vi "Callback - Get Data by Name.vi"(5 "Newest Time to Plot (unix,ns)":u64, 7 "Oldest Time to Plot (unix,ns)":u64, 8 "error in (no error)":errorcluster, 10 "Name":string, 11 "StokePlotHandle in":refnum<class "BjusticePlotHandle.lvclass">) -> (0 "error out":errorcluster, 2 "data history":T1, 3 "StokePlotHandle out":refnum<class "BjusticePlotHandle.lvclass">)   [LabVIEW 2021, in "BjusticePlotHandle.lvclass"]
uses:
  BjusticePlotHandle.lvclass
  TypeDefs/plot datapoint.ctl
  BjusticePlotHandle.lvclass/BjusticePlotHandle.ctl
  e8c38722-4420-420d-a7ba-0e160a98b42c.vi
  e8c38722-4420-420d-a7ba-0e160a98b42c.vi/17d75e1a-130a-47e0-8f2c-6c7d90b8ca77.vi
  <userlib>/bjustice/Ring Buffer for Time Series Data/API Poly.vi
  <userlib>/bjustice/Ring Buffer for Time Series Data/API/Read Full Rotated Buffer.vi
  <userlib>/bjustice/Ring Buffer for Time Series Data Strict Accessor/SubVIs/Search for time to keep.vi
  <userlib>/bjustice/Ring Buffer for Time Series Data Strict Accessor/SubVIs/Index ByteArray.vi
  e8c38722-4420-420d-a7ba-0e160a98b42c.vi/19bdd28a-0674-4be3-87bb-ec701e431d75.vi
  <userlib>/bjustice/Ring Buffer for Time Series Data Strict Accessor/SubVIs/error if empty buffer.vi
  e8c38722-4420-420d-a7ba-0e160a98b42c.vi/17d75e1a-130a-47e0-8f2c-6c7d90b8ca77.vi/bbb64351-fa28-4ac1-b583-44e271193ecd.vi
  <userlib>/bjustice/Ring Buffer for Time Series Data/SubVIs/Rotate Buffer.vi
  <userlib>/bjustice/Ring Buffer for Time Series Data Strict Accessor/SubVIs/Search for oldest time to keep.vi
  <userlib>/bjustice/Ring Buffer for Time Series Data Strict Accessor/SubVIs/Search for newest time to keep.vi
  <userlib>/bjustice/Ring Buffer for Time Series Data Strict Accessor/SubVIs/datatype byte size.vi
  <userlib>/bjustice/Ring Buffer for Time Series Data Strict Accessor/SubVIs/array sizes to number of points.vi
  e8c38722-4420-420d-a7ba-0e160a98b42c.vi/19bdd28a-0674-4be3-87bb-ec701e431d75.vi/81c66277-30bd-484c-9c7c-9646f36721bb.vi
  e8c38722-4420-420d-a7ba-0e160a98b42c.vi/19bdd28a-0674-4be3-87bb-ec701e431d75.vi/7ca10173-70f1-4bfb-9c4b-948090662032.vi
  e8c38722-4420-420d-a7ba-0e160a98b42c.vi/19bdd28a-0674-4be3-87bb-ec701e431d75.vi/ea4aced9-3494-4b3f-b998-02af6afbdac4.vi
  e8c38722-4420-420d-a7ba-0e160a98b42c.vi/19bdd28a-0674-4be3-87bb-ec701e431d75.vi/022c581c-5349-49df-98f9-5a038829ee63.vi
  e8c38722-4420-420d-a7ba-0e160a98b42c.vi/19bdd28a-0674-4be3-87bb-ec701e431d75.vi/ed40bcc8-bbaa-4b61-9e1a-b4b75cf21b06.vi
  e8c38722-4420-420d-a7ba-0e160a98b42c.vi/19bdd28a-0674-4be3-87bb-ec701e431d75.vi/f4b703c2-aaab-40a0-b3da-b0c22dc82d50.vi
  e8c38722-4420-420d-a7ba-0e160a98b42c.vi/19bdd28a-0674-4be3-87bb-ec701e431d75.vi/1efa054f-b143-4d96-9f7e-584a7c6fa7fd.vi
  e8c38722-4420-420d-a7ba-0e160a98b42c.vi/19bdd28a-0674-4be3-87bb-ec701e431d75.vi/b7c29f3f-256a-4401-af9d-aa15374df391.vi
  e8c38722-4420-420d-a7ba-0e160a98b42c.vi/19bdd28a-0674-4be3-87bb-ec701e431d75.vi/2fb7b479-974d-4a18-8674-c4c8d9dc9a89.vi
  e8c38722-4420-420d-a7ba-0e160a98b42c.vi/19bdd28a-0674-4be3-87bb-ec701e431d75.vi/faac7175-5814-4bb6-a961-a8db1f460653.vi
  e8c38722-4420-420d-a7ba-0e160a98b42c.vi/19bdd28a-0674-4be3-87bb-ec701e431d75.vi/b6af2a6f-71a4-4cfe-837f-b196861458b0.vi
  <userlib>/bjustice/Ring Buffer for Time Series Data/SubVIs/Split Values Array.vi
  <userlib>/bjustice/Ring Buffer for Time Series Data/SubVIs/Enforce array size multiple timestamps.vi
  <vilib>/Utility/error.llb/Trim Whitespace.vi
  <vilib>/Utility/error.llb/Error Cluster From Error Code.vi
  RocketPlot.lvlib
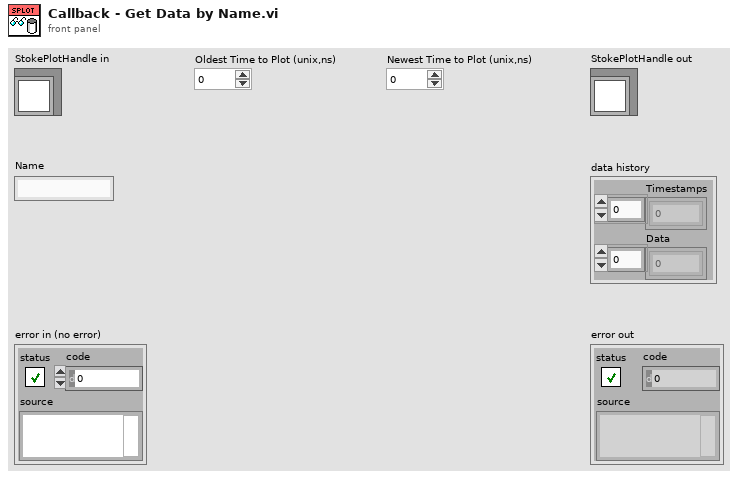
[diagram p1: front panel]
types:
  T1 = typedef "RocketPlot.lvlib/plot datapoint.ctl" = cluster{"Timestamps":u64[], "Data":dbl[]}
  T2 = typedef "Ring Buffer Strict Accessor.lvlib/RingBufferHandle.ctl" = cluster{"Ring buffer DVR":refnum<data-value>, "Data Type":T3, "Size(s)":i32[], "Endianess":T4, "Buffer Size (#timestamps) [init]":i32}
  T3 = typedef "Ring Buffer Strict Accessor.lvlib/DataType.ctl" = enum16{"uint8", "uint16", "uint32", "uint64", "int8", "int16", "int32", "int64", "float", "double", "extended"}
  T4 = typedef "Ring Buffer Strict Accessor.lvlib/Endianess.ctl" = enum16{"big-endian", "little-endian"}
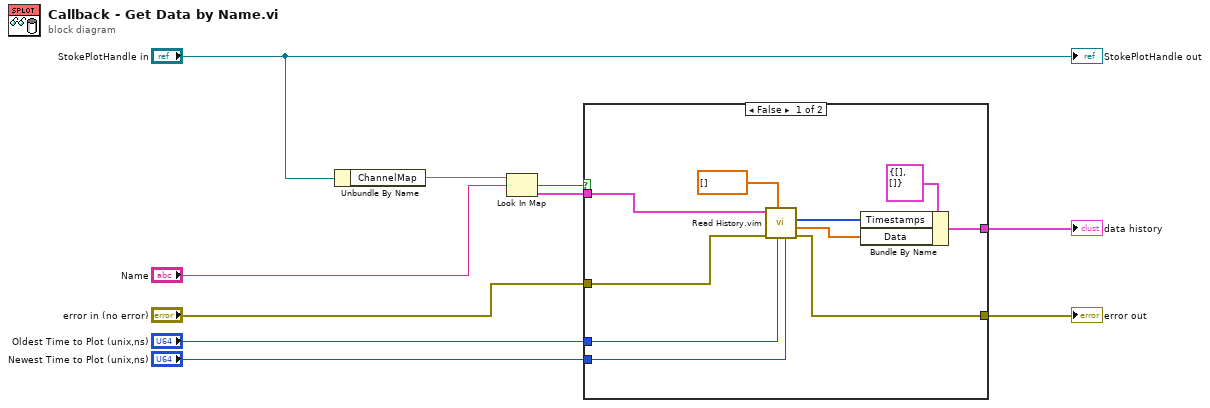
[diagram p0: block diagram]
diagram:
  n1 = Unbundle By Name("StokePlotHandle in") -> ("ChannelMap"=w6:map{string, T2})
  n2 = Look In Map(map=w6, key="Name") -> (key not found?=w5:bool, value=w4:T2)  [unwired: 1 in]
  n3 = case shown="False" w5 {
    tunnel: w4 -> [w13 _]
    tunnel: "Oldest Time to Plot (unix,ns)" -> [w15 _]
    tunnel: [w19 _] -> w10
    tunnel: "Newest Time to Plot (unix,ns)" -> [w14 _]
    tunnel: "error in (no error)" -> [w12 w21]
    tunnel: [w11 w21] -> w3
    frame False {
      n4 = call "Read History.vim"("newest time to keep"=w14, "oldest time to keep"=w15, "data type"=dbl[] [], "error in (no error)"=w12, "Ring Buffer"=w13) -> ("error out"=w11:errorcluster, "Values"=w17:dbl[], "Timestamps"=w18:u64[])  [unwired: 3 in, 1 out]
      n5 = Bundle By Name(cluster=T1 {"Timestamps"=[], "Data"=[]} ("data history"), "Timestamps"=w18, "Data"=w17) -> (w19:T1)
    }
    frame True {
    }
  }
  "error out" <- w3
  "data history" <- w10
  "StokePlotHandle out" <- "StokePlotHandle in"
